vi "command_line_output.vi"(10 "CMD Error":refnum<vi>, 11 "CMD Output":refnum<vi>) -> ()   [LabVIEW 2019]
panel:
  out "Standart Output":string
  out "Standart Error":string
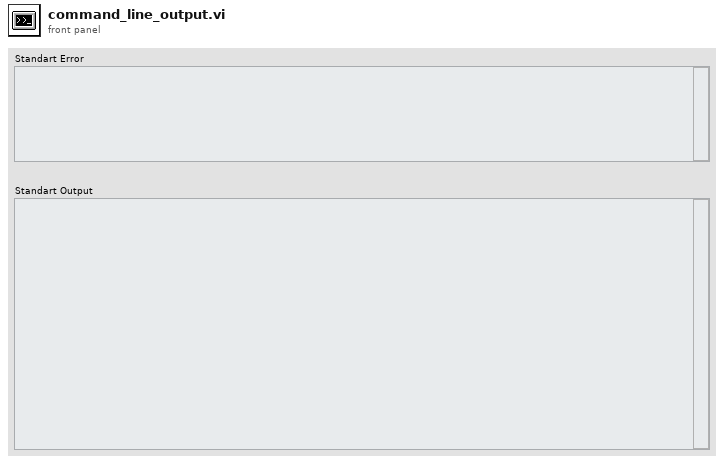
[diagram p1: front panel]
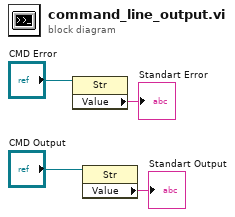
[diagram p0: block diagram]
diagram:
  n1 = property class="Str"(reference="CMD Error") -> ("Value"=→"Standart Error":string)  [unwired: 1 in, 2 out]
  n2 = property class="Str"(reference="CMD Output") -> ("Value"=→"Standart Output":string)  [unwired: 1 in, 2 out]
